vi "Control Car.vi"(8 "error in (no error)":errorcluster, 9 "Throttle":sgl, 10 "Steering":sgl, 11 "FormulaG API in":refnum<class "FormulaG API.lvclass">) -> (0 "error out":errorcluster, 3 "FormulaG API out":refnum<class "FormulaG API.lvclass">)   [LabVIEW 2020, in "FormulaG.lvlib" / "FormulaG API.lvclass"]
uses:
  FormulaG API.lvclass
  FormulaG-Common/Car Control.ctl
  Command.ctl
  FormulaG API.lvclass/FormulaG API.ctl
  FormulaG-Common/FormulaG-Common.lvlib
  <vilib>/IlluminatedG/IG GodotServer/GodotLV/GodotServer/GodotServer.lvclass
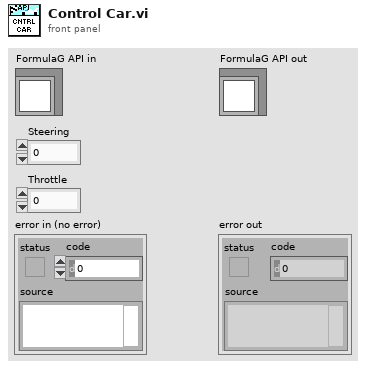
[diagram p1: front panel]
types:
  T1 = typedef "FormulaG.lvlib/FormulaG API.lvclass/Command.ctl" = enum8{"None", "Reset Car", "Request Ranges", "Control Car", "Request Info", "Set Options", "Set Camera", "Set Pause", "Request Time"}
  T2 = enum16{"big-endian, network order", "native, host order", "little-endian"}
  T3 = typedef "FormulaG-Common.lvlib/Car Control.ctl" = cluster{"Steering (-1 to 1)":sgl, "Throttle (0 to 1)":sgl}
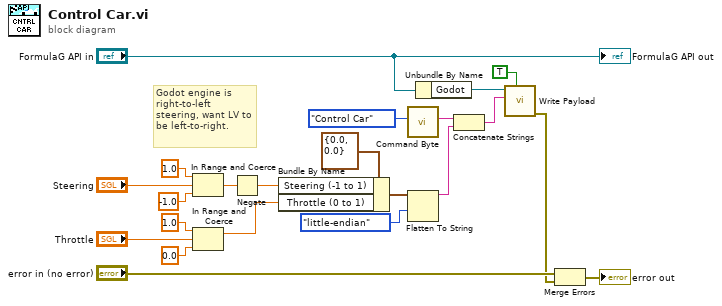
[diagram p0: block diagram]
diagram:
  # "Godot engine is right-to-left steering, want LV to be left-to-right."
  n1 = In Range and Coerce(upper limit=sgl 1.0, x="Steering", lower limit=sgl -1.0) -> (coerced(x)=w11:sgl)  [unwired: 1 out]
  n2 = In Range and Coerce(upper limit=sgl 1.0, x="Throttle", lower limit=sgl 0.0) -> (coerced(x)=w5:sgl)  [unwired: 1 out]
  n3 = Negate(x=w11) -> (-x=w19:sgl)
  n4 = Bundle By Name(cluster=T3 {"Steering (-1 to 1)"=0.0, "Throttle (0 to 1)"=0.0} ("Car Control"), "Steering (-1 to 1)"=w19, "Throttle (0 to 1)"=w5) -> (w17:T3)
  n5 = call "Command Byte.vi"("Command"=Command."Control Car") -> ("Command Byte"=w14:string)  [unwired: 10 in]
  n6 = Flatten To String(anything=w17, byte order (0:big-endian, network order)=T2."little-endian") -> (data string=w18:string)  [unwired: 2 in, 2 out]
  n7 = Unbundle By Name("FormulaG API in") -> ("Godot"=w4:refnum<class "GodotServer.lvclass">)
  n8 = Concatenate Strings(w14, w18) -> (w2:string)
  n9 = call <vilib>:"Write Payload.vi"("Binary (F = Text)"=TRUE, "Payload"=w2, "GodotServer in"=w4) -> ("error out"=w3:errorcluster)  [unwired: 7 in, 1 out]
  n10 = Merge Errors("error in (no error)", w3) -> (→"error out":errorcluster)
  "FormulaG API out" <- "FormulaG API in"
